vi "Format into Annotation BBox (SubVI).vi"(11 "Bounding Box":i32[](array[numeric])) -> (3 "Array":i32[](array[numeric]))   [LabVIEW 2015]
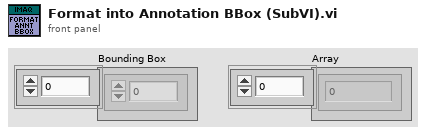
[diagram p1: front panel]
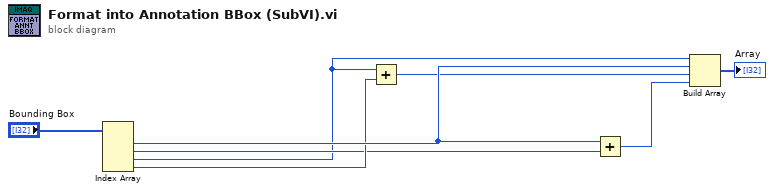
[diagram p0: block diagram]
diagram:
  n1 = Index Array(array="Bounding Box") -> (element #1=w5:i32, element #2=w2:i32, element #3=w1:i32, element #4=w3:i32)  [unwired: 4 in]
  n2 = Add(x=w1, y=w3) -> (x+y=w4:i32)
  n3 = Add(x=w5, y=w2) -> (x+y=w6:i32)
  n4 = Build Array(w1, w5, w4, w6) -> (→"Array":i32[])
